vi "FTW-File-CalculateRelativeFilepath.vi"(0 "Paths":path[](array[path]), 5 "Base Path":path) -> (4 "Relative Paths":path[](array[path]))   [LabVIEW 2012]
panel:
  # "Inputs"
  # "Outputs"
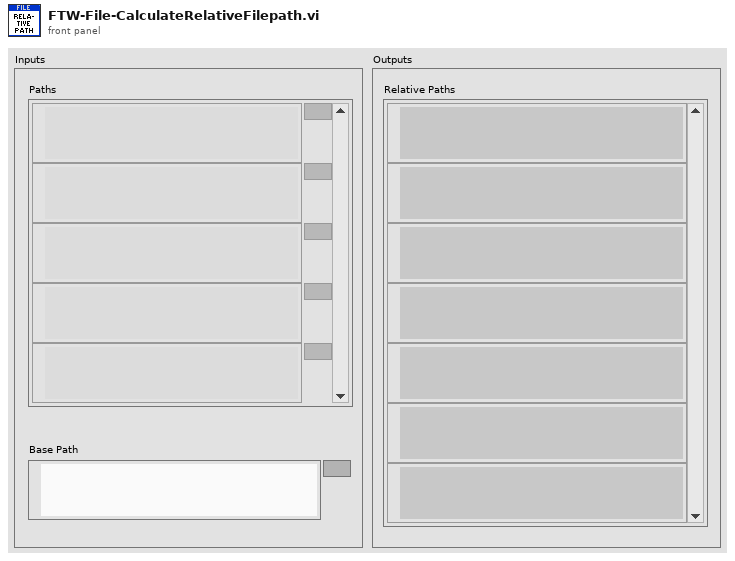
[diagram p1: front panel]
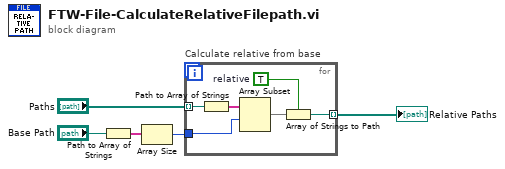
[diagram p0: block diagram]
diagram:
  n1 = Path to Array of Strings(0:"Base Path") -> (2:w5:string[])  [unwired: 1 out]
  n2 = Array Size(array=w5) -> (size(s)=w4:i32)
  n3 = for "Calculate relative from base" {
    tunnel: "Paths" -> [w11] mode=indexing
    tunnel: w4 -> [w9]
    tunnel: [w6] -> w2 mode=indexing
    w8 = TRUE  # relative
    n4 = Path to Array of Strings(0:w11) -> (2:w10:string[])  [unwired: 1 out]
    n5 = Array Subset(array=w10, index=w9) -> (w7:string[])  [unwired: 1 in]
    n6 = Array of Strings to Path(0:w7, 1:w8) -> (2:w6:path)
  }
  "Relative Paths" <- w2
